vi "New.vi"(8 "Error In":errorcluster, 10 "Old Delimiters":T1={"Close"="}}", "Open"="{{"}, 11 "New Delimiters":cluster{"Close":string, "Open":string}={"Close"="<%", "Open"="%>"}) -> (0 "Error Out":errorcluster, 3 "SetDelimiter":refnum<class "SetDelimiter.lvclass">)   [LabVIEW 2018, in "Toolkit.lvlib" / "Tokens.lvlib" / "SetDelimiter.lvclass"]
uses:
  SetDelimiter.lvclass
  Type Definitions/Delimiters.ctl
  SetDelimiter.lvclass/SetDelimiter.ctl
  Toolkit.lvlib
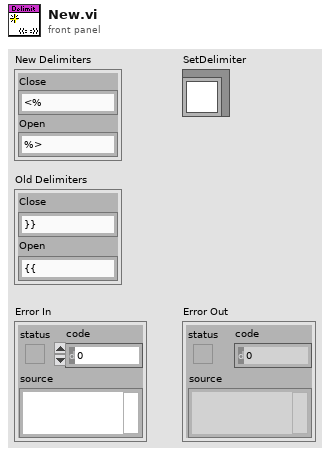
[diagram p1: front panel]
types:
  T1 = typedef "Toolkit.lvlib/Delimiters.ctl" = cluster{"Close":string, "Open":string}
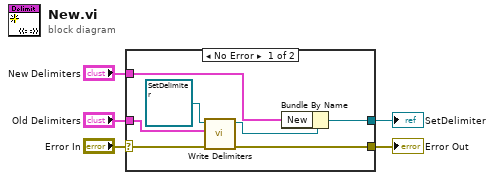
[diagram p0: block diagram]
diagram:
  n1 = case shown="No Error" "Error In" {
    selector: "Error In" -> [w6 w13]
    tunnel: [w12 w13] -> w5
    tunnel: "Old Delimiters" -> [w9 _]
    tunnel: [w8 _] -> w3
    tunnel: "New Delimiters" -> [w7 _]
    frame No Error {
      n2 = call-dynamic "Write Delimiters.vi"("Error In"=w6, "Delimiters"=w9, "Token In"=refnum<class "SetDelimiter.lvclass"> refnum ("Toolkit.lvlib:Tokens.lvlib:SetDelimiter.lvclass")) -> ("Error Out"=w12:errorcluster, "Token Out"=w10:refnum<class "SetDelimiter.lvclass">)  [unwired: 7 in]
      n3 = Bundle By Name(cluster=w10, "New"=w7) -> (w8:refnum<class "SetDelimiter.lvclass">)
    }
    frame Error {
    }
  }
  "Error Out" <- w5
  "SetDelimiter" <- w3
